vi "Scan Engine RemIO Module Page.vi"(8 "error in (no error)":errorcluster, 11 "Node Ptr":T1 format="%.0x") -> (0 "error out":errorcluster)   [LabVIEW 2015, in "Scan Engine Custom Device.lvlib"]
uses:
  Scan Engine Custom Device.lvlib
  <vilib>/NI Veristand/Custom Device API/Custom Device Item Ref.ctl
  Modules.lvlibp/RSI Module/SubPanel Command.ctl
  <vilib>/NI Veristand/Custom Device API/Custom Device API.lvlib
  Modules.lvlibp/RSI Module/RSI Module.lvclass
panel:
  in  "Header":cluster{"Section Name":string}={"Section Name"="Module Settings"}
  in  "Description":string
  out "Name":string
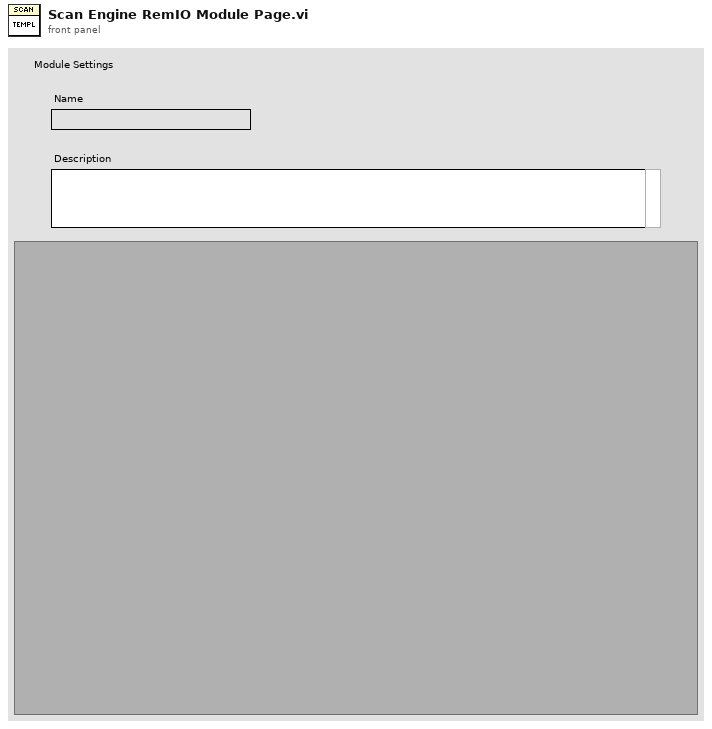
[diagram p1: front panel]
types:
  T1 = typedef "Custom Device API.lvlib/Custom Device Item Ref.ctl" = u64
  T2 = typedef "Custom Device API.lvlib/Custom Device Item Info.ctl" = cluster{"Name":string, "Is Channel":bool, "GUID":string, "Is Waveform":bool}
  T3 = typedef "Modules.lvlibp/RSI Module.lvclass/SubPanel Command.ctl" = enum16{"Stop"}
  T4 = typedef "Custom Device API.lvlib/Custom Device Commands.ctl" = enum16{"Default", "Item renamed", "Shutdown", "Dynamic button pressed"}
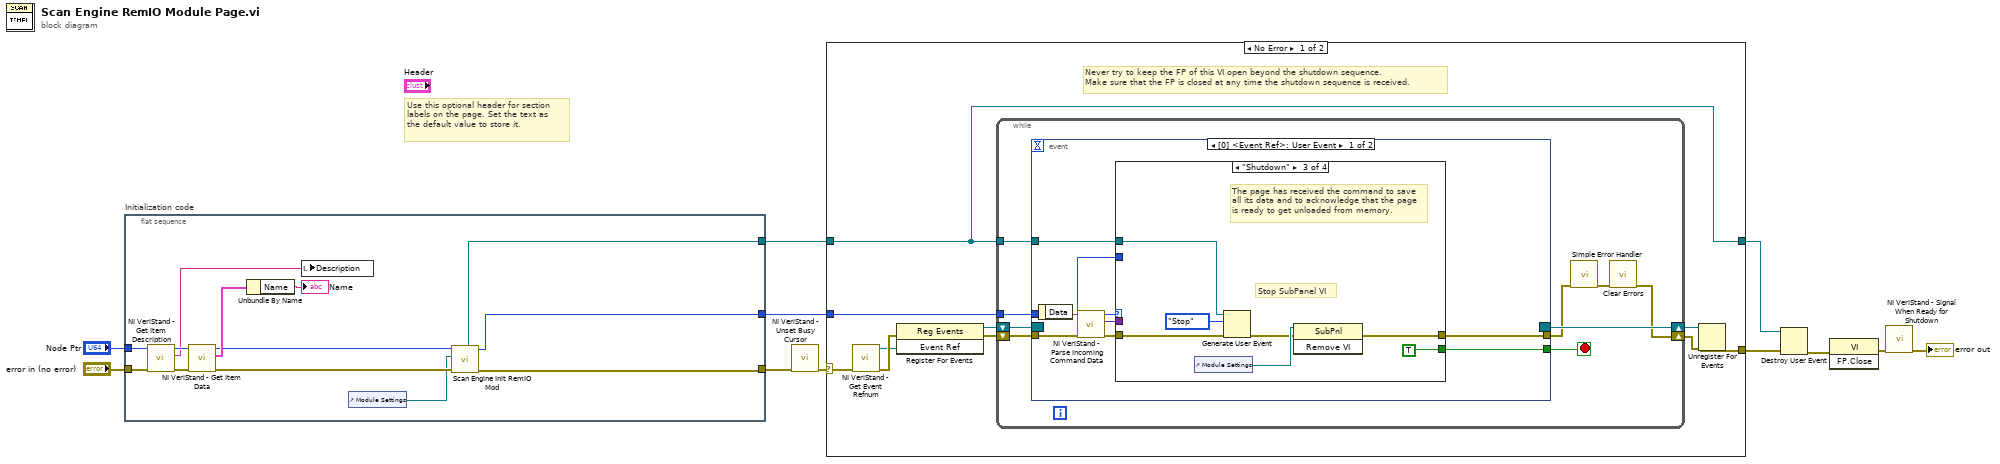
[diagram p0: block diagram]
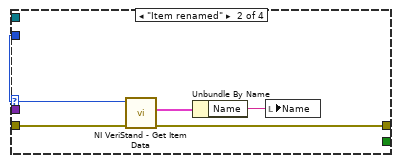
[diagram p3: hidden frame]
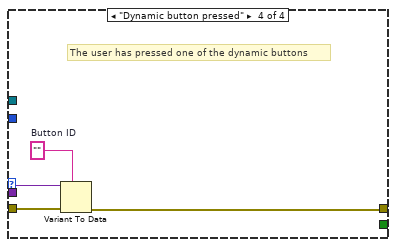
[diagram p4: hidden frame]
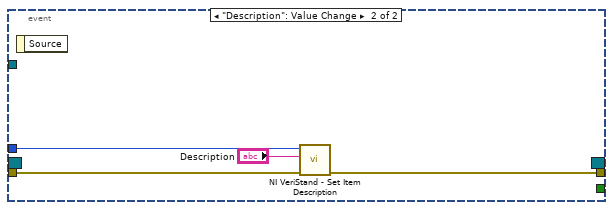
[diagram p5: hidden frame]
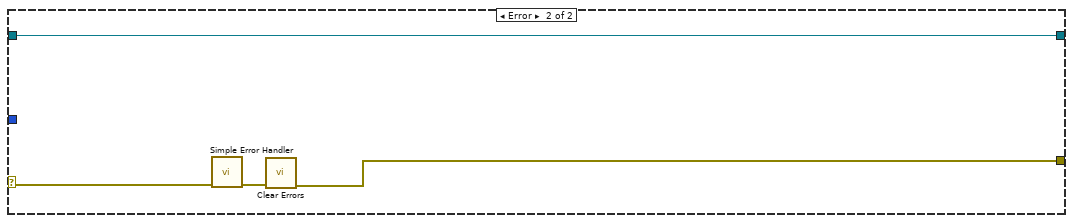
[diagram p6: hidden frame]
diagram:
  # "Use this optional header for section labels on the page. Set the text as the default value to store it."
  n1 = flat-sequence "Initialization code" {
    tunnel: "error in (no error)" -> [w18]
    tunnel: "Node Ptr" -> [w19]
    tunnel: [w12] -> w8
    tunnel: [w17] -> w5
    tunnel: [w13] -> w4
    frame #0 {
      n2 = call <vilib>:"NI VeriStand - Get Item Description.vi"("error in (no error)"=w18, "Item Ref in"=w19) -> ("error out"=w22:errorcluster, "Description"=w23:string, "Item Ref out"=w24:T1)  [unwired: 7 out]
      n3 = call <vilib>:"NI VeriStand - Get Item Data.vi"("error in (no error)"=w22, "Item Ref in"=w24) -> ("error out"=w15:errorcluster, "Item Info"=w21:T2, "Item Ref out"=w16:T1)  [unwired: 7 out]
      n4 = Unbundle By Name(w21) -> ("Name"=→"Name":string)
      n5 = local write "Description"(w23) -> ()
      n6 = control-ref of="Module Settings"() -> (w14:refnum<vi>)
      n7 = call "Scan Engine Init RemIO Mod.vi"("error in (no error)"=w15, "SubPanel Ref"=w14, "Node Ptr In"=w16) -> ("error out"=w12:errorcluster, "Node Ptr Out"=w17:T1, "SubPanel Command"=w13:refnum<user-event>)  [unwired: 6 in]
    }
  }
  n8 = call <vilib>:"NI VeriStand - Unset Busy Cursor.vi"("error in (no error)"=w8) -> ("error out"=w7:errorcluster)  [unwired: 10 out]
  n9 = case shown="No Error" w7 {
    selector: w7 -> [w26 w77]
    tunnel: [w31 w75] -> w2
    tunnel: w5 -> [w27 _]
    tunnel: w4 -> [w25 w74]
    tunnel: [w25 w74] -> w3
    frame No Error {
      # "Never try to keep the FP of this VI open beyond the shutdown sequence.\nMake sure that the FP is closed at any time the shutdown sequence is received."
      n10 = call <vilib>:"NI VeriStand - Get Event Refnum.vi"("error in (no error)"=w26) -> ("error out"=w34:errorcluster, "Event Ref"=w30:refnum<user-event>)  [unwired: 9 out]
      n11 = register-events(error in=w34, w30) -> (reference out=w28:refnum<event-registration>, error out=w29:errorcluster)  [unwired: 1 in]
      n12 = while {
        tunnel: w27 -> [w39]
        shift-right: [w36] -> w32
        shift-left: w29 -> [w42]
        shift-right: [w43] -> w33
        shift-left: w28 -> [w41]
        tunnel: w25 -> [w35]
        stop <- w40 stop-if-true
        n13 = event shown="[0] <Event Ref>: User Event" {
          selector: w41 -> [_ _]
          dyn-events: [_ _] -> w43
          timeout: _ -> [_ _]
          tunnel: w42 -> [w52 w72]
          tunnel: [w48 _] -> w40
          tunnel: [w47 w71] -> w38
          tunnel: w39 -> [w46 w73]
          tunnel: w35 -> [w44 _]
          event User Event {
            n14 = event-data() -> ("Data"=w51:string)  [unwired: 1 out]
            n15 = call <vilib>:"NI VeriStand - Parse Incoming Command Data.vi"("error in (no error)"=w52, "Incoming data"=w51) -> ("error out"=w50:errorcluster, "Outgoing data"=w45:variant, "Action"=w49:T4)  [unwired: 7 out]
            n16 = case shown="\"Shutdown\"" w49 {
              tunnel: w50 -> [w53 w58 w62 w69]
              tunnel: [_ _ TRUE _] -> w48
              tunnel: [w53 w55 w59 w66] -> w47
              tunnel: w46 -> [_ w57 _ _]
              tunnel: w45 -> [_ _ _ w68]
              tunnel: w44 -> [_ _ w64 _]
              frame "Default", Default {
              }
              frame "Item renamed" {
                n17 = call <vilib>:"NI VeriStand - Get Item Data.vi"("error in (no error)"=w58, "Item Ref in"=w57) -> ("error out"=w55:errorcluster, "Item Info"=w56:T2)  [unwired: 8 out]
                n18 = Unbundle By Name(w56) -> ("Name"=w54:string)
                n19 = local write "Name"(w54) -> ()
              }
              frame "Shutdown" {
                # "Stop SubPanel VI"
                # "The page has received the command to save all its data and to acknowledge that the page is ready to get unloaded from memory."
                n20 = control-ref of="Module Settings"() -> (w61:refnum<vi>)
                n21 = Generate User Event(user event=w64, event data cluster=SubPanel_Command."Stop" ("event data"), error in=w62) -> (error out=w60:errorcluster)  [unwired: 1 in, 1 out]
                n22 = invoke class="SubPnl" method="Remove VI"(reference=w61, error in=w60) -> (error out=w59:errorcluster)  [unwired: 1 in, 2 out]
              }
              frame "Dynamic button pressed" {
                w67 = ""  # Button ID
                # "The user has pressed one of the dynamic buttons"
                n23 = Variant To Data(error in=w69, type=w67, Variant=w68) -> (error out=w66:errorcluster)  [unwired: 1 out]
              }
            }
          }
          event "Description": Value Change {
            n24 = event-data() -> ()  [unwired: 2 out]
            n25 = call <vilib>:"NI VeriStand - Set Item Description.vi"("error in (no error)"=w72, "Description"="Description", "Item Ref in"=w73) -> ("error out"=w71:errorcluster)  [unwired: 8 out]
          }
        }
        n26 = call <vilib>:"Simple Error Handler.vi"("error in (no error)"=w38) -> ("error out"=w37:errorcluster)  [unwired: 1 in, 7 out]
        n27 = call <vilib>:"Clear Errors.vi"("error in (no error)"=w37) -> ("error out"=w36:errorcluster)  [unwired: 1 in, 5 out]
      }
      n28 = Unregister For Events(event registration refnum=w33, error in=w32) -> (error out=w31:errorcluster)
    }
    frame Error {
      n29 = call <vilib>:"Simple Error Handler.vi"("error in (no error)"=w77) -> ("error out"=w76:errorcluster)  [unwired: 1 in, 7 out]
      n30 = call <vilib>:"Clear Errors.vi"("error in (no error)"=w76) -> ("error out"=w75:errorcluster)  [unwired: 1 in, 5 out]
    }
  }
  n31 = Destroy User Event(user event=w3, error in=w2) -> (error out=w1:errorcluster)
  n32 = invoke class="VI" method="FP.Close"(error in=w1) -> (error out=w11:errorcluster)  [unwired: 2 in, 2 out]
  n33 = call <vilib>:"NI VeriStand - Signal When Ready for Shutdown.vi"("error in (no error)"=w11) -> ("error out"=→"error out":errorcluster)  [unwired: 10 out]
